vi "AppendToMarkers.vi"(8 "Owner":u8=255, 9 "Color":u32(colorbox)=32639, 10 "Pixels 3":dbl[][](array[numeric]), 11 "MarkersArray":T1) -> (0 "Owner Out":u8=255, 3 "MarkersArray Out":T1)   [LabVIEW 2017, in "ImageAcquisitionLibrary.lvlib"]
uses:
  ImageAcquisitionLibrary.lvlib
  MarkersArray.ctl
  Marker.ctl
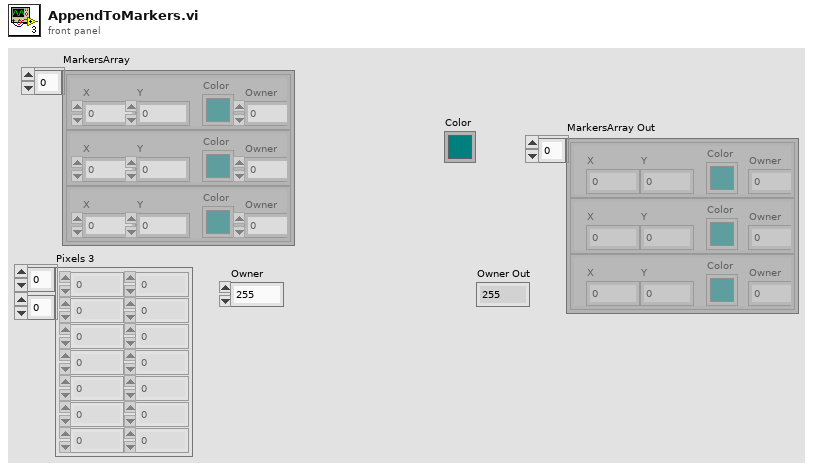
[diagram p1: front panel]
types:
  T1 = typedef "ImageAcquisitionLibrary.lvlib/MarkersArray.ctl" = T2[]
  T2 = typedef "ImageAcquisitionLibrary.lvlib/Marker.ctl" = cluster{"X":dbl, "Color":u32, "Y ":dbl, "Owner":u8}
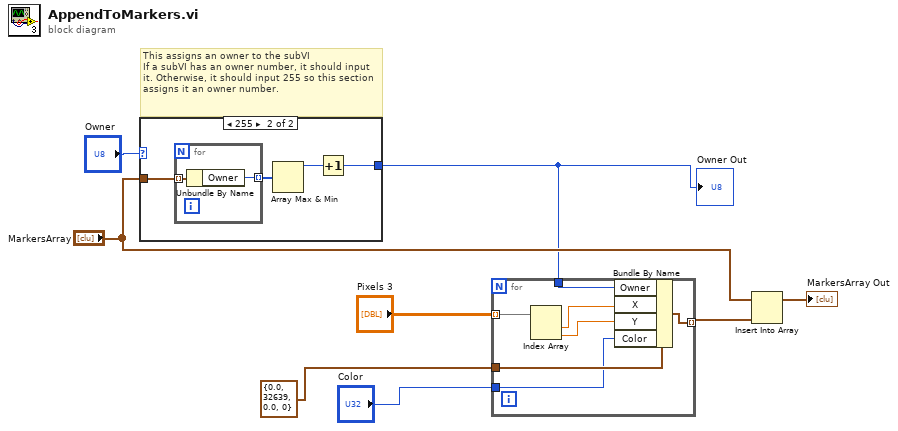
[diagram p0: block diagram]
diagram:
  # "This assigns an owner to the subVI\nIf a subVI has an owner number, it should input it. Otherwise, it should input 255 so this section assigns it an owner number."
  n1 = case shown="255" "Owner" {
    selector: "Owner" -> [w9 _]
    tunnel: "MarkersArray" -> [_ w13]
    tunnel: [w9 w10] -> w1
    frame 0, Default {
    }
    frame 255 {
      n2 = for {
        tunnel: w13 -> [w15] mode=indexing
        tunnel: [w14] -> w12 mode=indexing
        n3 = Unbundle By Name(w15) -> ("Owner"=w14:u8)
      }
      n4 = Array Max & Min(array=w12) -> (max value=w11:u8)  [unwired: 3 out]
      n5 = Increment(x=w11) -> (x+1=w10:u8)
    }
  }
  "Owner Out" <- w1
  n6 = for {
    tunnel: "Pixels 3" -> [w21] mode=indexing
    tunnel: T2 {"X"=0.0, "Color"=32639, "Y "=0.0, "Owner"=0} ("Marker") -> [w22]
    tunnel: "Color" -> [w18]
    tunnel: [w17] -> w6 mode=indexing
    tunnel: w1 -> [w16]
    n7 = Index Array(array=w21) -> (element #1=w20:dbl, element #2=w19:dbl)  [unwired: 2 in]
    n8 = Bundle By Name(cluster=w22, "Owner"=w16, "X"=w20, "Y"=w19, "Color"=w18) -> (w17:T2)
  }
  n9 = Insert Into Array(array="MarkersArray", new element=w6) -> (→"MarkersArray Out":T1)  [unwired: 1 in]
